vi "Frame Ready.vi"(8 "error in (no error)":errorcluster, 9 "Processed Frames per Second":dbl, 10 "Image In":T1, 11 "CameraComm in":refnum<class "CameraComm.lvclass">) -> (0 "error out":errorcluster, 3 "CameraComm out":refnum<class "CameraComm.lvclass">)   [LabVIEW 2023, in "CameraComm.lvlib" / "CameraComm.lvclass"]
uses:
  CameraComm.lvclass
  <vilib>/vision/Image Controls.llb/IMAQ Image.ctl
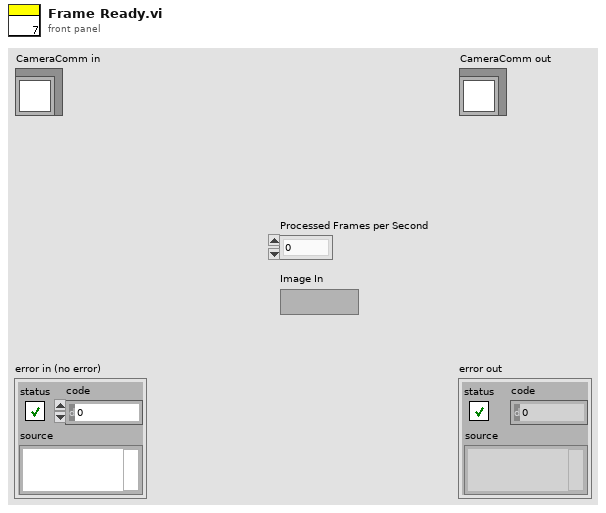
[diagram p1: front panel]
types:
  T1 = typedef "IMAQ Image.ctl" = refnum<image>
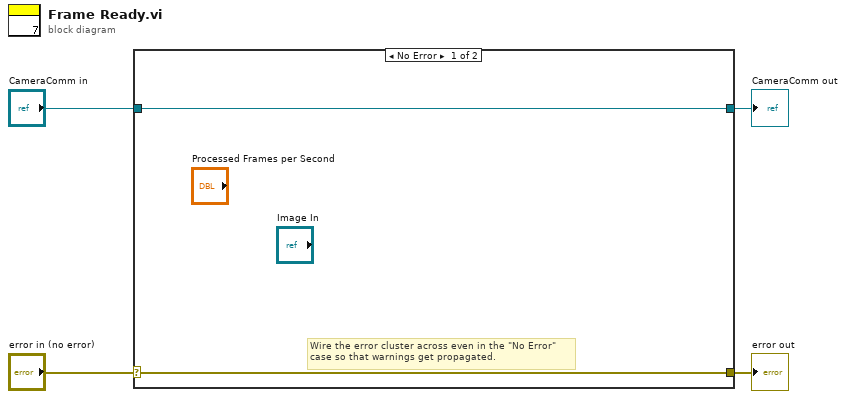
[diagram p0: block diagram]
diagram:
  n1 = case shown="No Error" "error in (no error)" {
    selector: "error in (no error)" -> [w5 w8]
    tunnel: [w5 w8] -> w3
    tunnel: [w6 w7] -> w1
    tunnel: "CameraComm in" -> [w6 w7]
    frame No Error {
      # "Wire the error cluster across even in the \"No Error\"\ncase so that warnings get propagated."
    }
    frame Error {
    }
  }
  "error out" <- w3
  "CameraComm out" <- w1
